vi "[FPGA] HIL_DECC_CRios_ES2 Controller with comm_clean up version_1229.vi"() -> ()   [LabVIEW 2015]
uses:
  2015 SP1 Support Files/IP Cores/IP Cores - LabVIEW FPGA/Control & Signal Gen/Controls/PID Float Simple Multichannel Channel Configuration.ctl
  <vilib>/rvi/Emulation/niFpgaGetClockAttributes.vi
  <vilib>/rvi/Emulation/niFpgaSctlEmulationGetInTimedLoop.vi
  <vilib>/rvi/Emulation/niFpgaEmulationReportErrorSimple.vi
  <vilib>/rvi/Emulation/niFpgaProcessEmulError.vi
  2015 SP1 Support Files/IP Cores/IP Cores - LabVIEW FPGA/Floating Point/Polymorphic subVIs/Multiply 00.vi
  2015 SP1 Support Files/IP Cores/IP Cores - LabVIEW FPGA/Floating Point/Polymorphic subVIs/Add 00.vi
  2015 SP1 Support Files/IP Cores/IP Cores - LabVIEW FPGA/Floating Point/Polymorphic subVIs/Subtract 00.vi
  <vilib>/rvi/Emulation/niFpgaCriticalErrorInLSC.vi
  <vilib>/rvi/eio/common/nirviEmuTemplateMethod_errors.vi
  2015 SP1 Support Files/IP Cores/IP Cores - LabVIEW FPGA/Floating Point/Polymorphic subVIs/Divide 00.vi
  2015 SP1 Support Files/IP Cores/IP Cores - LabVIEW FPGA/Floating Point/Polymorphic subVIs/Square 00.vi
  2015 SP1 Support Files/IP Cores/IP Cores - LabVIEW FPGA/Floating Point/Polymorphic subVIs/Absolute Value 00.vi
  <vilib>/eio/EIONode/EIONode.xnode
panel:
  out "PLL_phase":sgl
  in  "I scale":sgl[](array[numeric])=[40.0, 0.0, 0.0]
  in  "V scale":sgl[](array[numeric])=[100.0, 0.0, 0.0]
  in  "LTYPE":sgl=1.0
  in  "dt (s)":sgl=7.5e-05
  in  "reinitialize? (F)":bool
  in  "Debounce (iterations)":i32=5
  out "Power Analysis":T1(array[cluster])
  out "Power Analysis\n loop time":u32
  in  "Phase Offset":sgl=-0.5235988 format="%.16g"
  out "Verror":sgl
  out "PLL_sin(x)":sgl
  in  "range":cluster{"upper limit":sgl, "lower limit":sgl}={"upper limit"=70.0, "lower limit"=45.0}
  in  "PLL dt":sgl=0.001
  in  "reference F":sgl=50.0
  in  "PLL PI gains":T2={"proportional gain (Kp)"=10.0, "integral gain (Ki)"=2.0}
  in  "V Control Params":T3[](array[typedef])=[{"Write Channel"=TRUE, "Channel #"=2, "dt (s)"=0.0001, "Kp"=0.25, "Ki [Hz]"=5.0, "Kd [Hz]"=0.0, "upper limit"=200.0, "lower limit"=-200.0, "LPF alpha"=0.018}, {"Write Channel"=TRUE, "Channel #"=3, "dt (s)"=0.0001, "Kp"=0.25, "Ki [Hz]"=5.0, "Kd [Hz]"=0.0, "upper limit"=200.0, "lower limit"=-200.0, "LPF alpha"=0.018}] {"Kp" step=0.125}
  in  "I Control Params":T3[](array[typedef])=[{"Write Channel"=TRUE, "Channel #"=0, "dt (s)"=0.0001, "Kp"=0.01, "Ki [Hz]"=0.1, "Kd [Hz]"=0.0, "upper limit"=2.5, "lower limit"=-2.5, "LPF alpha"=0.018}, {"Write Channel"=TRUE, "Channel #"=1, "dt (s)"=0.0001, "Kp"=0.01, "Ki [Hz]"=0.1, "Kd [Hz]"=0.0, "upper limit"=2.5, "lower limit"=-2.5, "LPF alpha"=0.018}] {"Kp" step=0.125}
  out "Fault Cluster":T4
  out "Fault":bool
  in  "Clear Fault":bool
  in  "Over V ignore":bool
  in  "V_max":sgl=470.0
  in  "Over I ignore":bool
  in  "I_max":sgl=150.0
  in  "Vrms_min":fxp<+,24,8>=2.449951171875
  in  "I^2_max":sgl=10000.0
  in  "Vdc_min":sgl=770.0
  in  "Vdc_max":sgl=970.0
  out "Vf Control_Enabled":bool
  out "Q_ES":sgl
  in  "PI Reset":bool
  out "Vc":fxp<+/-,24,5> format="%.21g"
  out "Vb":fxp<+/-,24,5> format="%.21g"
  out "Va":fxp<+/-,24,5> format="%.21g"
  out "Ic":fxp<+/-,24,5> format="%.21g"
  out "Ib":fxp<+/-,24,5> format="%.21g"
  out "Ia":fxp<+/-,24,5> format="%.21g"
  out "Vc RMS":sgl format="%.2f"
  out "Vb RMS":sgl format="%.2f"
  out "Va RMS":sgl format="%.2f"
  in  "Droop_Qmax":sgl=20000.0
  in  "Droop Enabled":bool
  in  "Vf Control_ES":bool
  in  "PWM Enable_ES":bool
  in  "2*islanded (s)":fxp<+,30,1>=3.999099135398865e-06
  in  "islanded (us)":u32=6
  out "islanded (uSec)":u32=24763547
  out "phase reset":bool
  in  "AI Rate (Ticks)":u32=3000
  out "SOC%":fxp<+/-,24,5>=-0.000339508056640625 format="%.21g"
  out "Vb_Microgrid":sgl=0.004022043 format="%.2f"
  out "f":fxp<+,20,6>=2.0 format="%.27g"
  out "phase_micro":fxp<+/-,32,1> format="%.32g"
  in  "f_resyn":fxp<+,20,6>=60.050048828125 format="%#_27g"
  in  "f_islanded":fxp<+,20,6>=60.0
  in  "Resyn_enable":bool
  out "control loop dt_ES":u32=100
  in  "P_ref_ES":sgl
  in  "L_ES":sgl=0.01
  out "Dd_ES":sgl=-0.19541435 format="%.2f"
  out "Dq_ES":sgl=-0.14656767 format="%.2f"
  out "Iq_ref_ES":sgl
  in  "Q_ref_ES":sgl
  in  "PQ Control_ES":bool
  in  "Id_setpoint_ES":sgl
  out "Id_ref_ES":sgl
  in  "Iq_setpoint_ES":sgl
  in  "Vq_setpoint_ES":sgl
  out "Qmeas_ES":sgl=4.594709e-05
  out "Pmeas_ES":sgl=-0.00010936371
  out "Vq_ES":sgl=-0.0007594844
  out "Vd_ES":sgl=-0.0020615412
  out "Iq_ES":sgl=-0.0006459089 format="%.2f"
  out "Id_ES":sgl=0.0012190519 format="%.2f"
  out "Vabc_ES":sgl[](array[numeric])=[0.0053937677, 0.005342122, 0.0078376485] format="%.2f"
  in  "LPF Alpha_VolES":sgl[](array[numeric])=[0.19, 0.19, 0.19]
  in  "Vab_ES Gain":sgl=100.0
  out "Vavg_ES":sgl=6.7118024e-05
  out "Iabc_ES":sgl[](array[numeric])=[0.0054930565, -0.023219703, -0.0023527772] format="%.2f"
  in  "LPF Alpha_CurrES":sgl[](array[numeric])=[0.32, 0.32, 0.32, 0.01]
  in  "DC LPF enable":bool
  in  "LPF enable":bool=TRUE
  in  "Iinv Gain":sgl=40.0
  in  "Vdc Gain":sgl=200.0
  in  "stop":bool
  in  "time reset":bool
  out "freq_ES":sgl=2.0 format="%.2f"
  out "PLL dT (Ticks)":u32=3000
  out "sin(x)_ES":sgl=-6.1035156e-05 format="%.2f"
  out "cos(x)_ES":sgl=0.99993896 format="%.2f"
  out "AI dT (Ticks)":u32=3000
  # "Control Configuration"
  # "Loop Time"
  # "Low-pass Filters"
  # "Calibration"
  # "Data Display"
  # "Power Analysis"
  # "Control Loop Parameters"
  # "PLL Loop"
  # "Freq for VF Mode"
  # "Protection"
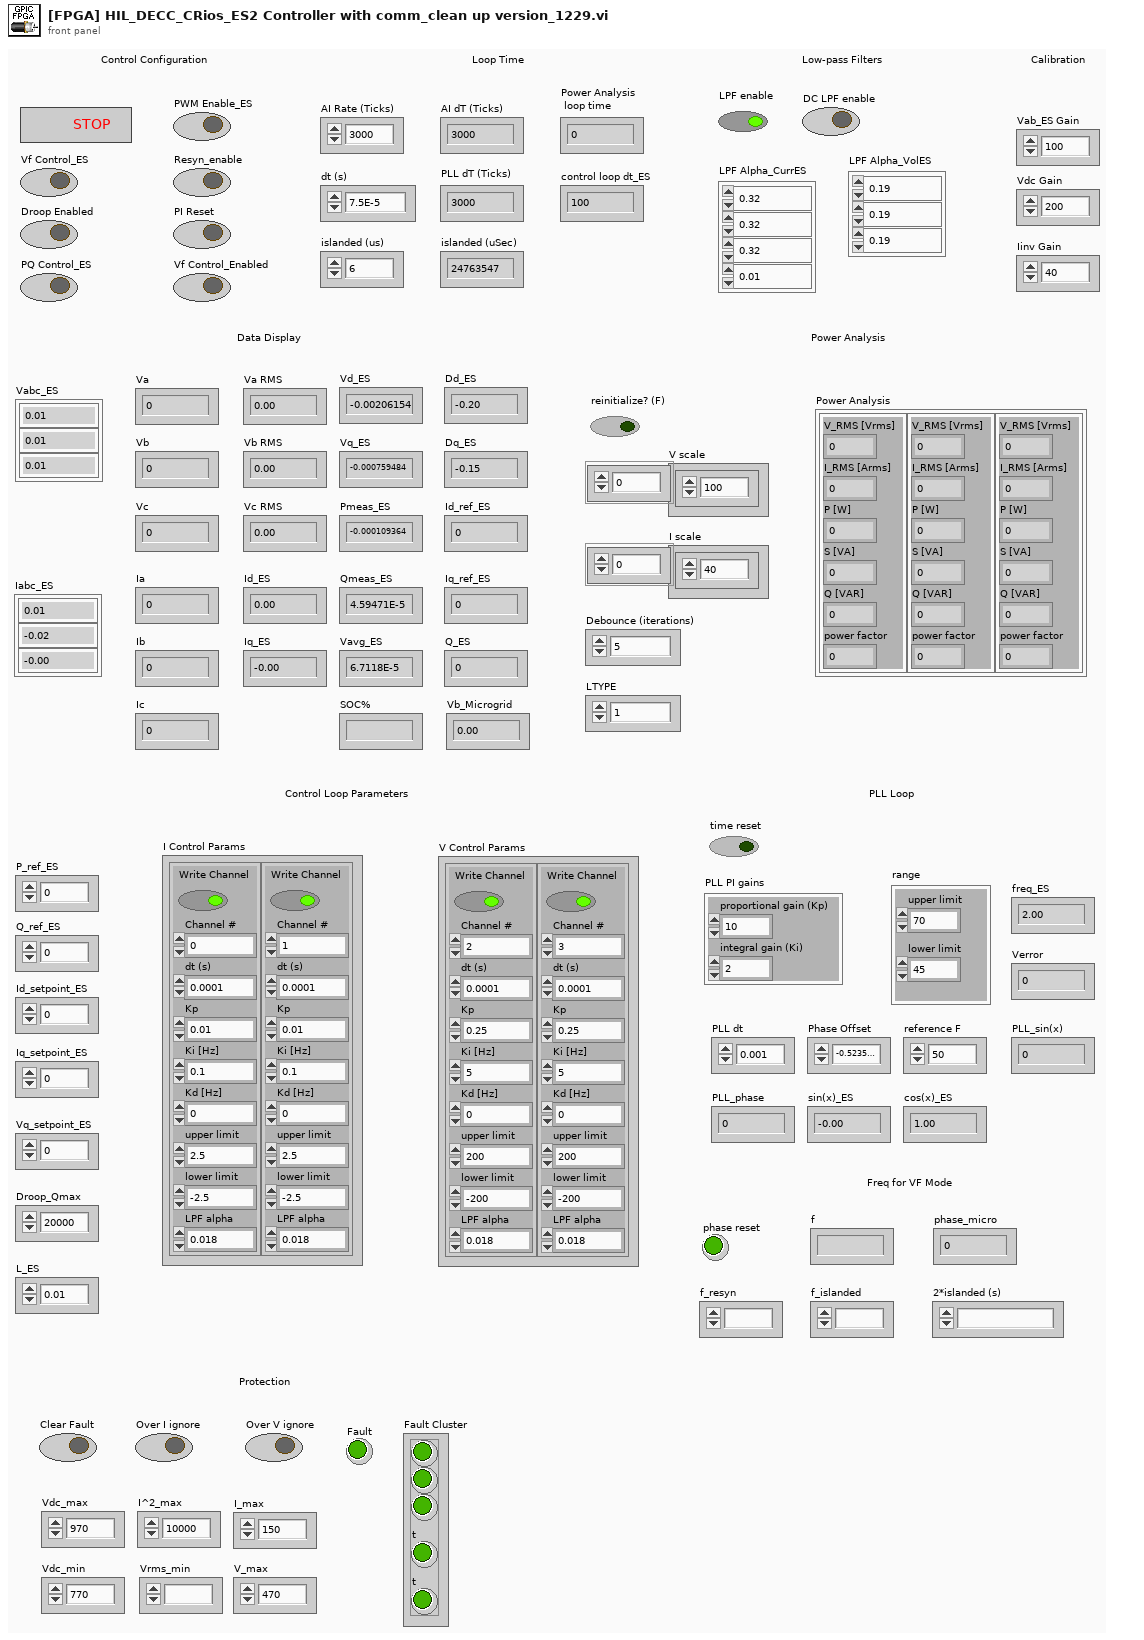
[diagram p1: front panel]
types:
  T1 = cluster{"V_RMS [Vrms] ":sgl, "I_RMS [Arms]":sgl, "P [W]":sgl, "S [VA]":sgl, "Q [VAR]":sgl, "power factor":sgl}[]
  T2 = cluster{"proportional gain (Kp)":sgl, "integral gain (Ki)":sgl}
  T3 = typedef "PID Float Simple Multichannel Channel Configuration.ctl" = cluster{"Write Channel":bool, "Channel #":u32, "dt (s)":sgl, "Kp":sgl, "Ki [Hz]":sgl, "Kd [Hz]":sgl, "upper limit":sgl, "lower limit":sgl, "LPF alpha":sgl}
  T4 = cluster{"Boolean":bool, "Boolean":bool, "Boolean":bool, "t":bool, "t":bool}
  T5 = cluster{"V_RMS [Vrms] ":sgl, "I_RMS [Arms]":sgl, "P [W]":sgl, "S [VA]":sgl, "Q [VAR]":sgl, "power factor":sgl}
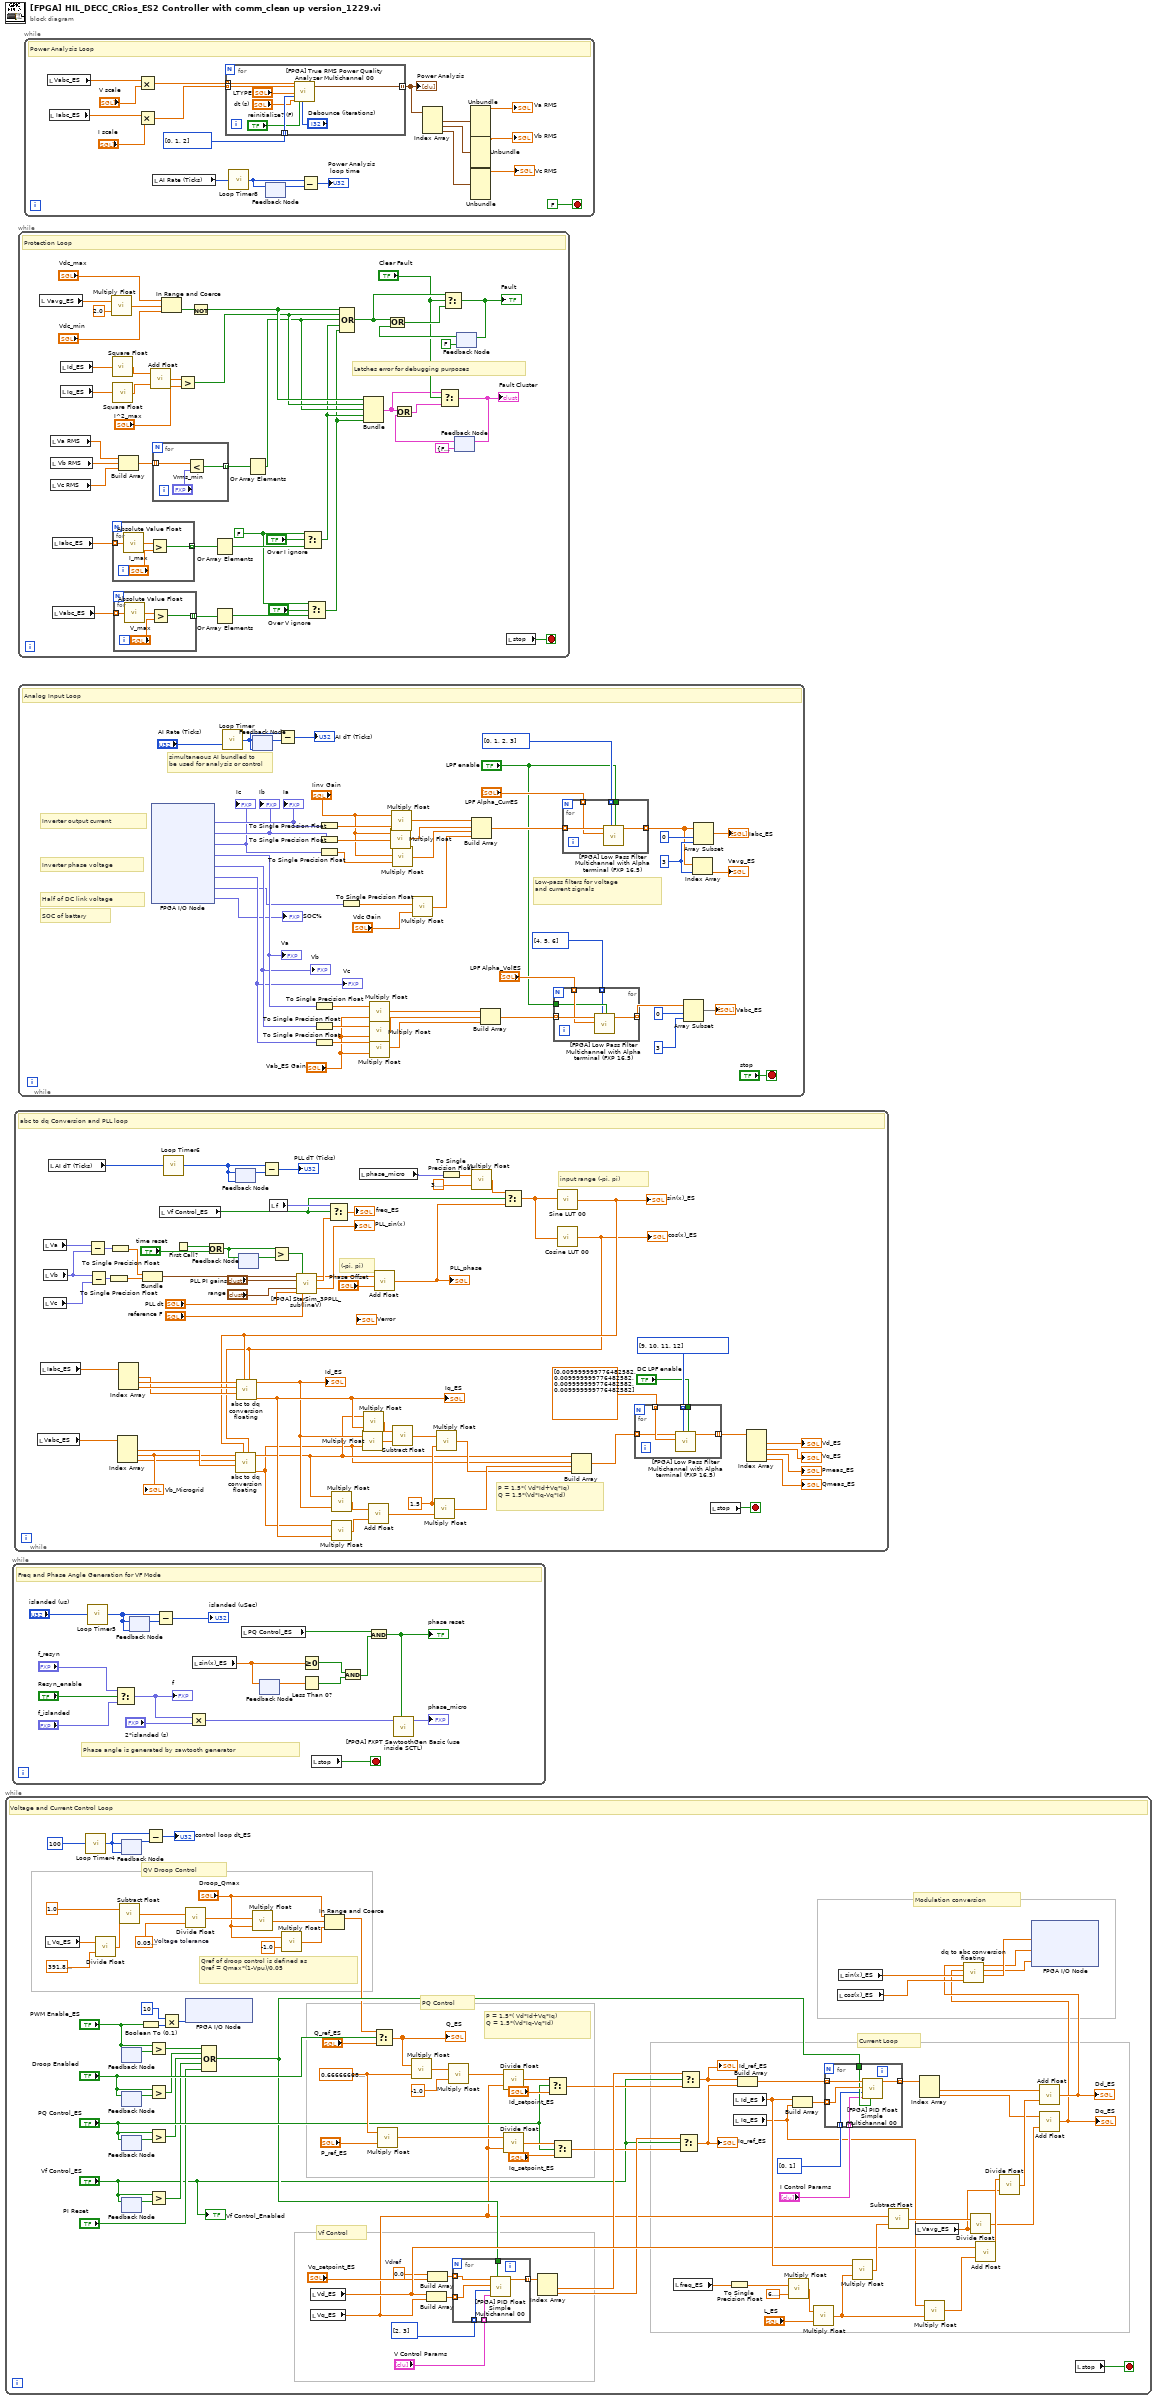
[diagram p0: block diagram]
diagram:
  n1 = while {
    stop <- w79 stop-if-true
    w16 = sgl 0.05  # Voltage tolerance
    w49 = sgl 0.0  # Vdref
    w35 = sgl 0.6666667 ("y")
    # "Modulation conversion"
    # "Current Loop"
    # "Vf Control"
    # "PQ Control"
    # "QV Droop Control"
    # "P = 1.5*( Vd*Id+Vq*Iq)\nQ = 1.5*(Vd*Iq-Vq*Id)"
    # "Qref of droop control is defined as\nQref = Qmax*(1-Vpu)/0.05"
    # "Voltage and Current Control Loop"
    n2 = local read "Vq_ES"() -> (w20:sgl)
    n3 = call "Loop Timer4"("Count(uSec)"=u32 100) -> ("Tick Count(uSec)"=w75:u32)
    n4 = call-poly "Divide Float.vi"("y"=sgl 391.9, "x"=w20) -> ("x/y"=w18:sgl)
    n5 = call-poly "Subtract Float.vi"("y"=w18, "x"=sgl 1.0) -> ("x*y"=w17:sgl)
    n6 = feedback #1(w75) -> (w88:u32)
    n7 = feedback-in #1(w75) -> ()
    n8 = feedback #2() -> (w29:bool)  [unwired: 1 in]
    n9 = feedback-in #2("PWM Enable_ES") -> ()
    n10 = feedback #3() -> (w31:bool)  [unwired: 1 in]
    n11 = feedback-in #3("Droop Enabled") -> ()
    n12 = feedback #4() -> (w33:bool)  [unwired: 1 in]
    n13 = feedback-in #4("PQ Control_ES") -> ()
    n14 = feedback #5() -> (w47:bool)  [unwired: 1 in]
    n15 = feedback-in #5("Vf Control_ES") -> ()
    n16 = Boolean To (0,1)(Boolean="PWM Enable_ES") -> (0, 1=w38:i16)
    n17 = Subtract(x=w75, y=w88) -> (x-y=→"control loop dt_ES":u32)
    n18 = Greater?(x="PWM Enable_ES", y=w29) -> (0:w27:bool)
    n19 = Greater?(x="Droop Enabled", y=w31) -> (0:w26:bool)
    n20 = Greater?(x="PQ Control_ES", y=w33) -> (0:w25:bool)
    n21 = Greater?(x="Vf Control_ES", y=w47) -> (0:w24:bool)
    n22 = Multiply(x=i16 10, y=w38) -> (x*y=w37:i16)
    n23 = call-poly "Divide Float.vi"("y"=w16, "x"=w17) -> ("x/y"=w15:sgl)
    n24 = xnode "FPGA I/O Node"("Mod4/AO3"=w37) -> ()  [unwired: 1 in, 1 out]
    n25 = Compound Arithmetic op=OR(w27, w26, w25, w24, "PI Reset") -> (w23:bool)
    n26 = call-poly "Multiply Float.vi"("y"="Droop_Qmax", "x"=w15) -> ("x*y"=w14:sgl)
    n27 = call-poly "Multiply Float.vi"("y"=sgl -1.0, "x"="Droop_Qmax") -> ("x*y"=w10:sgl)
    n28 = local read "Vd_ES"() -> (w51:sgl)
    n29 = local read "Vq_ES"() -> (w7:sgl)
    n30 = In Range and Coerce(upper limit="Droop_Qmax", x=w14, lower limit=w10) -> (coerced(x)=w13:sgl)  [unwired: 1 out]
    n31 = Select(t=w13, s="Droop Enabled", f="Q_ref_ES") -> (s? t:f=w9:sgl)
    "Q_ES" <- w9
    n32 = call-poly "Multiply Float.vi"("y"="P_ref_ES", "x"=w35) -> ("x*y"=w64:sgl)
    n33 = call-poly "Multiply Float.vi"("y"=w35, "x"=w9) -> ("x*y"=w65:sgl)
    n34 = Build Array(w51, w7) -> (w54:sgl[])
    n35 = Build Array(w49, "Vq_setpoint_ES") -> (w53:sgl[])
    n36 = call-poly "Multiply Float.vi"("y"=sgl -1.0, "x"=w65) -> ("x*y"=w73:sgl)
    n37 = for {
      tunnel: [w96] -> w52 mode=indexing
      tunnel: w53 -> [w93] mode=indexing
      tunnel: w54 -> [w95] mode=indexing
      tunnel: i8[] [2, 3] ("appended array") -> [w94] mode=indexing
      tunnel: w23 -> [w92]
      tunnel: "V Control Params" -> [w91] mode=indexing
      n38 = call "[FPGA] PID Float Simple Multichannel 00.vi"("reinitialize? (F)"=w92, "Channel Config."=w91, "Channel #"=w94, "Process Variable"=w95, "Setpoint"=w93) -> ("Output"=w96:sgl)  [unwired: 4 in, 2 out]
    }
    n39 = call-poly "Divide Float.vi"("y"=w7, "x"=w73) -> ("x/y"=w72:sgl)
    n40 = call-poly "Divide Float.vi"("y"=w7, "x"=w64) -> ("x/y"=w70:sgl)
    n41 = Index Array(array=w52) -> (element #1=w43:sgl, element #2=w41:sgl)  [unwired: 2 in]
    n42 = Select(t=w72, s="PQ Control_ES", f="Id_setpoint_ES") -> (s? t:f=w42:sgl)
    n43 = Select(t=w70, s="PQ Control_ES", f="Iq_setpoint_ES") -> (s? t:f=w40:sgl)
    n44 = local read "freq_ES"() -> (w90:sgl)
    n45 = Select(t=w41, s="Vf Control_ES", f=w40) -> (s? t:f=w55:sgl)
    "Iq_ref_ES" <- w55
    n46 = Select(t=w43, s="Vf Control_ES", f=w42) -> (s? t:f=w56:sgl)
    "Id_ref_ES" <- w56
    n47 = To Single Precision Float(number=w90) -> (single precision float=w78:sgl)
    n48 = local read "Id_ES"() -> (w61:sgl)
    n49 = local read "Iq_ES"() -> (w2:sgl)
    n50 = Build Array(w56, w55) -> (w62:sgl[])
    n51 = call-poly "Multiply Float.vi"("y"=sgl 6.2831855, "x"=w78) -> ("x*y"=w86:sgl)
    n52 = Build Array(w61, w2) -> (w60:sgl[])
    n53 = call-poly "Multiply Float.vi"("y"="L_ES", "x"=w86) -> ("x*y"=w1:sgl)
    n54 = for {
      tunnel: [w102] -> w63 mode=indexing
      tunnel: w62 -> [w101] mode=indexing
      tunnel: w60 -> [w100] mode=indexing
      tunnel: w23 -> [w99]
      tunnel: i8[] [0, 1] ("appended array") -> [w98] mode=indexing
      tunnel: "I Control Params" -> [w97] mode=indexing
      n55 = call "[FPGA] PID Float Simple Multichannel 00.vi"("reinitialize? (F)"=w99, "Channel Config."=w97, "Channel #"=w98, "Process Variable"=w100, "Setpoint"=w101) -> ("Output"=w102:sgl)  [unwired: 4 in, 2 out]
    }
    n56 = local read "cos(x)_ES"() -> (w76:sgl)
    n57 = local read "sin(x)_ES"() -> (w77:sgl)
    n58 = call-poly "Multiply Float.vi"("y"=w1, "x"=w61) -> ("x*y"=w84:sgl)
    n59 = call-poly "Subtract Float.vi"("y"=w84, "x"=w7) -> ("x*y"=w83:sgl)
    n60 = local read "Vavg_ES"() -> (w48:sgl)
    n61 = Index Array(array=w63) -> (element #1=w58:sgl, element #2=w57:sgl)  [unwired: 2 in]
    n62 = call-poly "Multiply Float.vi"("y"=w1, "x"=w2) -> ("x*y"=w85:sgl)
    n63 = call-poly "Divide Float.vi"("y"=w48, "x"=w83) -> ("x/y"=w81:sgl)
    n64 = call-poly "Add Float.vi"("y"=w85, "x"=w51) -> ("x+y"=w82:sgl)
    n65 = call-poly "Divide Float.vi"("y"=w48, "x"=w82) -> ("x/y"=w80:sgl)
    n66 = call-poly "Add Float.vi"("y"=w80, "x"=w58) -> ("x+y"=w45:sgl)
    "Dd_ES" <- w45
    n67 = call-poly "Add Float.vi"("y"=w81, "x"=w57) -> ("x+y"=w44:sgl)
    "Dq_ES" <- w44
    n68 = call "dq to abc conversion floating.vi"("cos"=w76, "sin"=w77, "q"=w44, "d"=w45) -> ("c"=w68:sgl, "b"=w66:sgl, "a"=w67:sgl)  [unwired: 5 in]
    n69 = xnode "FPGA I/O Node"("Mod4/AO0"=w68, "Mod4/AO1"=w67, "Mod4/AO2"=w66) -> ()  [unwired: 3 in, 3 out]
    n70 = local read "stop"() -> (w79:bool)
    "Vf Control_Enabled" <- "Vf Control_ES"
  }
  n71 = while {
    stop <- w121 stop-if-true
    # "Phase angle is generated by sawtooth generator"
    # "Freq and Phase Angle Generation for VF Mode"
    n72 = call "Loop Timer5"("Count(uSec)"="islanded (us)") -> ("Tick Count(uSec)"=w118:u32)
    n73 = Select(t="f_resyn", s="Resyn_enable", f="f_islanded") -> (s? t:f=w116:fxp<+,20,6>)
    "f" <- w116
    n74 = feedback #6(w118) -> (w119:u32)
    n75 = feedback-in #6(w118) -> ()
    n76 = Subtract(x=w118, y=w119) -> (x-y=→"islanded (uSec)":u32)
    n77 = Multiply(x=w116, y="2*islanded (s)") -> (x*y=w113:fxp<+,50,7>)
    n78 = local read "sin(x)_ES"() -> (w107:sgl)
    n79 = local read "PQ Control_ES"() -> (w109:bool)
    n80 = feedback #7() -> (w106:sgl)  [unwired: 1 in]
    n81 = feedback-in #7(w107) -> ()
    n82 = Greater Or Equal To 0?(x=w107) -> (x >= 0?=w104:bool)
    n83 = Less Than 0?(x=w106) -> (x < 0?=w105:bool)
    n84 = local read "stop"() -> (w121:bool)
    n85 = And(x=w104, y=w105) -> (x .and. y?=w103:bool)
    n86 = And(x=w109, y=w103) -> (x .and. y?=w108:bool)
    "phase reset" <- w108
    n87 = call "[FPGA] FXPT SawtoothGen Basic (use inside SCTL).vi"("reset (rising edge)"=w108, "Carrier Frequency (=fo(Hz)*2*dT)"=w113) -> ("Sawtooth"=→"phase_micro":fxp<+/-,32,1>)  [unwired: 9 in]
  }
  n88 = while {
    stop <- w188 stop-if-true
    w164 = sgl 1.5 ("x")
    # "(-pi, pi)"
    # "input range (-pi, pi)"
    # "P = 1.5*( Vd*Id+Vq*Iq)\nQ = 1.5*(Vd*Iq-Vq*Id)"
    # "abc to dq Conversion and PLL loop"
    n89 = local read "Vabc_ES"() -> (w174:sgl[])
    n90 = local read "Iabc_ES"() -> (w178:sgl[])
    n91 = local read "Va"() -> (w146:fxp<+/-,24,5>)
    n92 = local read "Vb"() -> (w144:fxp<+/-,24,5>)
    n93 = local read "Vc"() -> (w143:fxp<+/-,24,5>)
    n94 = local read "AI dT (Ticks)"() -> (w180:u32)
    n95 = Subtract(x=w146, y=w144) -> (x-y=w145:fxp<+/-,25,6>)
    n96 = Subtract(x=w144, y=w143) -> (x-y=w142:fxp<+/-,25,6>)
    n97 = To Single Precision Float(number=w142) -> (single precision float=w140:sgl)
    n98 = To Single Precision Float(number=w145) -> (single precision float=w141:sgl)
    n99 = Index Array(array=w174) -> (element #1=w149:sgl, element #2=w148:sgl, element #3=w147:sgl)  [unwired: 3 in]
    "Vb_Microgrid" <- w148
    n100 = Index Array(array=w178) -> (element #1=w175:sgl, element #2=w177:sgl, element #3=w176:sgl)  [unwired: 3 in]
    n101 = Bundle(w141, w140) -> (w139:cluster{sgl, sgl})  [unwired: 1 in]
    n102 = local read "Vf Control_ES"() -> (w150:bool)
    n103 = call "Loop Timer6"("Count(Ticks)"=w180) -> ("Tick Count(Ticks)"=w186:u32)
    n104 = First Call?() -> (First Call?: T/F=w184:bool)
    n105 = Or(x=w184, y="time reset") -> (x .or. y?=w182:bool)
    n106 = feedback #8(w186) -> (w187:u32)
    n107 = feedback-in #8(w186) -> ()
    n108 = feedback #9() -> (w181:bool)  [unwired: 1 in]
    n109 = feedback-in #9(w182) -> ()
    n110 = Subtract(x=w186, y=w187) -> (x-y=→"PLL dT (Ticks)":u32)
    n111 = local read "f"() -> (w151:fxp<+,20,6>)
    n112 = Greater?(x=w182, y=w181) -> (0:w138:bool)
    n113 = call "[FPGA] StarSim_3PPLL_sub(lineV).vi"("phase voltage"=w139, "reset"=w138, "PI gains"="PLL PI gains", "range"="range", "dt"="PLL dt", "reference F"="reference F") -> ("phase x"=w131:sgl, "frequency"=w132:sgl, "sin(x)"=→"PLL_sin(x)":sgl)  [unwired: 4 in, 3 out]
    n114 = Select(t=w151, s=w150, f=w132) -> (s? t:f=→"freq_ES":sgl)
    n115 = local read "phase_micro"() -> (w128:fxp<+/-,32,1>)
    n116 = call-poly "Add Float.vi"("y"="Phase Offset", "x"=w131) -> ("x+y"=w129:sgl)
    "PLL_phase" <- w129
    n117 = To Single Precision Float(number=w128) -> (single precision float=w127:sgl)
    n118 = call-poly "Multiply Float.vi"("y"=sgl 3.1415927, "x"=w127) -> ("x*y"=w125:sgl)
    n119 = Select(t=w125, s=w150, f=w129) -> (s? t:f=w122:sgl)
    n120 = call "Sine LUT 00.vi"("x"=w122) -> ("sin(x)"=w124:sgl)
    "sin(x)_ES" <- w124
    n121 = call "Cosine LUT 00.vi"("x"=w122) -> ("sin(x)"=w123:sgl)
    "cos(x)_ES" <- w123
    n122 = call "abc to dq conversion floating.vi"("cos"=w123, "sin"=w124, "C"=w149, "B"=w147, "A"=w148) -> ("q"=w161:sgl, "d"=w162:sgl)  [unwired: 5 in]
    n123 = call "abc to dq conversion floating.vi"("cos"=w123, "sin"=w124, "C"=w175, "B"=w176, "A"=w177) -> ("q"=w169:sgl, "d"=w168:sgl)  [unwired: 5 in]
    "Id_ES" <- w168
    "Iq_ES" <- w169
    n124 = call-poly "Multiply Float.vi"("y"=w168, "x"=w162) -> ("x*y"=w173:sgl)
    n125 = call-poly "Multiply Float.vi"("y"=w169, "x"=w161) -> ("x*y"=w172:sgl)
    n126 = call-poly "Multiply Float.vi"("y"=w161, "x"=w168) -> ("x*y"=w166:sgl)
    n127 = call-poly "Multiply Float.vi"("y"=w169, "x"=w162) -> ("x*y"=w167:sgl)
    n128 = call-poly "Add Float.vi"("y"=w172, "x"=w173) -> ("x+y"=w171:sgl)
    n129 = call-poly "Subtract Float.vi"("y"=w166, "x"=w167) -> ("x*y"=w165:sgl)
    n130 = call-poly "Multiply Float.vi"("y"=w171, "x"=w164) -> ("x*y"=w170:sgl)
    n131 = call-poly "Multiply Float.vi"("y"=w164, "x"=w165) -> ("x*y"=w163:sgl)
    n132 = Build Array(w162, w161, w170, w163) -> (w158:sgl[])
    n133 = for {
      tunnel: w158 -> [w190] mode=indexing
      tunnel: sgl[] [0.01, 0.01, 0.01, 0.01] ("DC LPF Alpha_ES") -> [w193] mode=indexing
      tunnel: [w192] -> w157 mode=indexing
      tunnel: u32[] [9, 10, 11, 12] -> [w191] mode=indexing
      tunnel: "DC LPF enable" -> [w189]
      n134 = call "[FPGA] Low Pass Filter Multichannel with Alpha terminal (FXP 16,5).vi"("enable"=w189, "Channel #"=w191, "LPF alpha"=w193, "x"=w190) -> ("filtered x"=w192:sgl)  [unwired: 7 in]
    }
    n135 = local read "stop"() -> (w188:bool)
    n136 = Index Array(array=w157) -> (element #1=→"Vd_ES":sgl, element #2=→"Vq_ES":sgl, element #3=→"Pmeas_ES":sgl, element #4=→"Qmeas_ES":sgl)  [unwired: 4 in]
  }
  n137 = while {
    stop <- w194 stop-if-true
    w211 = FALSE ("t")
    # "Latches error for debugging purposes"
    # "Protection Loop"
    n138 = local read "Vavg_ES"() -> (w236:sgl)
    n139 = local read "Va RMS"() -> (w224:sgl)
    n140 = local read "Vc RMS"() -> (w222:sgl)
    n141 = local read "Vb RMS"() -> (w223:sgl)
    n142 = local read "Vabc_ES"() -> (w215:sgl[])
    n143 = local read "Iabc_ES"() -> (w219:sgl[])
    n144 = local read "Id_ES"() -> (w230:sgl)
    n145 = local read "Iq_ES"() -> (w229:sgl)
    n146 = call-poly "Multiply Float.vi"("y"=sgl 2.0, "x"=w236) -> ("x*y"=w234:sgl)
    n147 = call-poly "Square Float.vi"("x"=w230) -> ("x^2"=w228:sgl)
    n148 = for {
      tunnel: w219 -> [w244] mode=indexing
      tunnel: [w241] -> w218 mode=indexing
      n149 = call-poly "Absolute Value Float.vi"("x"=w244) -> ("abs(x)"=w243:sgl)
      n150 = Greater?(x=w243, y="I_max") -> (0:w241:bool)
    }
    n151 = call-poly "Square Float.vi"("x"=w229) -> ("x^2"=w227:sgl)
    n152 = for {
      tunnel: w215 -> [w240] mode=indexing
      tunnel: [w237] -> w214 mode=indexing
      n153 = call-poly "Absolute Value Float.vi"("x"=w240) -> ("abs(x)"=w239:sgl)
      n154 = Greater?(x=w239, y="V_max") -> (0:w237:bool)
    }
    n155 = Build Array(w224, w223, w222) -> (w221:sgl[])
    n156 = call-poly "Add Float.vi"("y"=w227, "x"=w228) -> ("x+y"=w226:sgl)
    n157 = for {
      tunnel: w221 -> [w247] mode=indexing
      tunnel: [w245] -> w220 mode=indexing
      n158 = Less?(x=w247, y="Vrms_min") -> (x < y?=w245:bool)
    }
    n159 = In Range and Coerce(upper limit="Vdc_max", x=w234, lower limit="Vdc_min") -> (In Range?=w231:bool)  [unwired: 1 out]
    n160 = Greater?(x=w226, y="I^2_max") -> (0:w209:bool)
    n161 = Not(x=w231) -> (.not. x?=w210:bool)
    n162 = Or Array Elements(Boolean array=w218) -> (logical OR=w216:bool)
    n163 = Or Array Elements(Boolean array=w214) -> (logical OR=w213:bool)
    n164 = Or Array Elements(Boolean array=w220) -> (logical OR=w208:bool)
    n165 = Select(t=w211, s="Over I ignore", f=w216) -> (s? t:f=w207:bool)
    n166 = Select(t=w211, s="Over V ignore", f=w213) -> (s? t:f=w206:bool)
    n167 = Compound Arithmetic op=OR(w210, w209, w208, w207, w206) -> (w205:bool)
    n168 = Bundle(w210, w209, w208, "t"=w207, "t"=w206) -> (w199:cluster{bool, bool, bool, "t":bool, "t":bool})  [unwired: 1 in]
    n169 = feedback #10(cluster{bool, bool, bool, "t":bool, "t":bool} {FALSE, FALSE, FALSE, "t"=FALSE, "t"=FALSE}) -> (w196:cluster{bool, bool, bool, "t":bool, "t":bool})
    n170 = Or(x=w199, y=w196) -> (x .or. y?=w198:cluster{bool, bool, bool, "t":bool, "t":bool})
    n171 = Select(t=w199, s="Clear Fault", f=w198) -> (s? t:f=w197:cluster{bool, bool, bool, "t":bool, "t":bool})
    "Fault Cluster" <- w197
    n172 = feedback-in #10(w197) -> ()
    n173 = feedback #11(FALSE) -> (w202:bool)
    n174 = Or(x=w205, y=w202) -> (x .or. y?=w201:bool)
    n175 = Select(t=w205, s="Clear Fault", f=w201) -> (s? t:f=w204:bool)
    "Fault" <- w204
    n176 = feedback-in #11(w204) -> ()
    n177 = local read "stop"() -> (w194:bool)
  }
  n178 = while {
    stop <- "stop" stop-if-true
    w274 = 3 ("length")
    # "SOC of battary"
    # "Half of DC link voltage"
    # "Inverter phase voltage"
    # "Inverter output current"
    # "Low-pass filters for voltage \nand current signals"
    # "simultaneous AI bundled to\nbe used for analysis or control"
    # "Analog Input Loop"
    n179 = xnode "FPGA I/O Node"() -> ("Mod2/AI0"=w260:fxp<+/-,24,5>, "Mod2/AI1"=w259:fxp<+/-,24,5>, "Mod2/AI2"=w258:fxp<+/-,24,5>, "Mod2/AI3"=w257:fxp<+/-,24,5>, "Mod2/AI4"=w256:fxp<+/-,24,5>, "Mod2/AI5"=w255:fxp<+/-,24,5>, "Mod2/AI6"=w254:fxp<+/-,24,5>, "Mod2/AI7"=→"SOC%":fxp<+/-,24,5>)  [unwired: 8 in, 8 out]
    "Ia" <- w260
    "Ib" <- w259
    "Ic" <- w258
    "Va" <- w257
    "Vb" <- w256
    "Vc" <- w255
    n180 = call "Loop Timer"("Count(Ticks)"="AI Rate (Ticks)") -> ("Tick Count(Ticks)"=w292:u32)
    n181 = feedback #12(w292) -> (w291:u32)
    n182 = feedback-in #12(w292) -> ()
    n183 = Subtract(x=w292, y=w291) -> (x-y=→"AI dT (Ticks)":u32)
    n184 = To Single Precision Float(number=w257) -> (single precision float=w271:sgl)
    n185 = To Single Precision Float(number=w256) -> (single precision float=w270:sgl)
    n186 = To Single Precision Float(number=w255) -> (single precision float=w269:sgl)
    n187 = To Single Precision Float(number=w260) -> (single precision float=w288:sgl)
    n188 = To Single Precision Float(number=w259) -> (single precision float=w287:sgl)
    n189 = To Single Precision Float(number=w258) -> (single precision float=w286:sgl)
    n190 = To Single Precision Float(number=w254) -> (single precision float=w285:sgl)
    n191 = call-poly "Multiply Float.vi"("y"="Vab_ES Gain", "x"=w271) -> ("x*y"=w268:sgl)
    n192 = call-poly "Multiply Float.vi"("y"="Vab_ES Gain", "x"=w270) -> ("x*y"=w267:sgl)
    n193 = call-poly "Multiply Float.vi"("y"="Vab_ES Gain", "x"=w269) -> ("x*y"=w266:sgl)
    n194 = call-poly "Multiply Float.vi"("y"=w287, "x"="Iinv Gain") -> ("x*y"=w282:sgl)
    n195 = call-poly "Multiply Float.vi"("y"=w288, "x"="Iinv Gain") -> ("x*y"=w283:sgl)
    n196 = call-poly "Multiply Float.vi"("y"=w286, "x"="Iinv Gain") -> ("x*y"=w281:sgl)
    n197 = call-poly "Multiply Float.vi"("y"="Vdc Gain", "x"=w285) -> ("x*y"=w280:sgl)
    n198 = Build Array(w283, w282, w281, w280) -> (w279:sgl[])
    n199 = Build Array(w268, w267, w266) -> (w265:sgl[])
    n200 = for {
      tunnel: w265 -> [w298] mode=indexing
      tunnel: "LPF Alpha_VolES" -> [w297] mode=indexing
      tunnel: "LPF enable" -> [w296]
      tunnel: [w295] -> w248 mode=indexing
      tunnel: u32[] [4, 5, 6] -> [w294] mode=indexing
      n201 = call "[FPGA] Low Pass Filter Multichannel with Alpha terminal (FXP 16,5).vi"("enable"=w296, "Channel #"=w294, "LPF alpha"=w297, "x"=w298) -> ("filtered x"=w295:sgl)  [unwired: 7 in]
    }
    n202 = for {
      tunnel: w279 -> [w303] mode=indexing
      tunnel: "LPF Alpha_CurrES" -> [w302] mode=indexing
      tunnel: "LPF enable" -> [w301]
      tunnel: [w300] -> w273 mode=indexing
      tunnel: u32[] [0, 1, 2, 3] -> [w299] mode=indexing
      n203 = call "[FPGA] Low Pass Filter Multichannel with Alpha terminal (FXP 16,5).vi"("enable"=w301, "Channel #"=w299, "LPF alpha"=w302, "x"=w303) -> ("filtered x"=w300:sgl)  [unwired: 7 in]
    }
    n204 = Array Subset(array=w248, index=0, length=3) -> (→"Vabc_ES":sgl[])
    n205 = Index Array(array=w273, index=w274) -> (element=→"Vavg_ES":sgl)
    n206 = Array Subset(array=w273, index=0, length=w274) -> (→"Iabc_ES":sgl[])
  }
  n207 = while {
    stop <- FALSE stop-if-true
    # "Power Analysis Loop"
    n208 = local read "Vabc_ES"() -> (w315:sgl[])
    n209 = local read "Iabc_ES"() -> (w316:sgl[])
    n210 = Multiply(x=w315, y="V scale") -> (x*y=w313:sgl[])
    n211 = Multiply(x=w316, y="I scale") -> (x*y=w312:sgl[])
    n212 = local read "AI Rate (Ticks)"() -> (w318:u32)
    n213 = for {
      tunnel: w313 -> [w330] mode=indexing
      tunnel: [w329] -> w310 mode=indexing
      tunnel: w312 -> [w328] mode=indexing
      tunnel: u32[] [0, 1, 2] -> [w326] mode=indexing
      n214 = call "[FPGA] True RMS Power Quality Analyzer Multichannel 00.vi"("V [V]"=w330, "I [A]"=w328, "LTYPE"="LTYPE", "Channel #"=w326, "dt (s)"="dt (s)", "reinitialize? (F)"="reinitialize? (F)", "Debounce (iterations)"="Debounce (iterations)") -> ("Power Analysis"=w329:T5)  [unwired: 12 in]
    }
    "Power Analysis" <- w310
    n215 = call "Loop Timer8"("Count(Ticks)"=w318) -> ("Tick Count(Ticks)"=w319:u32)
    n216 = feedback #13() -> (w320:u32)  [unwired: 1 in]
    n217 = feedback-in #13(w319) -> ()
    n218 = Subtract(x=w319, y=w320) -> (x-y=→"Power Analysis\n loop time":u32)
    n219 = Index Array(array=w310) -> (element #1=w309:T5, element #2=w308:T5, element #3=w307:T5)  [unwired: 3 in]
    n220 = Unbundle(w309) -> ("V_RMS [Vrms]"=→"Va RMS":sgl)  [unwired: 5 out]
    n221 = Unbundle(w308) -> ("V_RMS [Vrms]"=→"Vb RMS":sgl)  [unwired: 5 out]
    n222 = Unbundle(w307) -> ("V_RMS [Vrms]"=→"Vc RMS":sgl)  [unwired: 5 out]
  }
